vi "CAN_Command Ford.vi"(5 "CAN Command":string, 6 "ID Response":string="18DAF255", 7 "Numeric Request":u32 format="%x", 8 "ID Request":string="18DA55F2", 9 "Read":refnum<k21>, 10 "Write":refnum<k21>) -> (0 "Data String":string, 1 "ID String":string, 2 "Write out":refnum<k21>, 3 "Read out":refnum<k21>, 4 "Timestamp":timestamp)   [LabVIEW 2023]
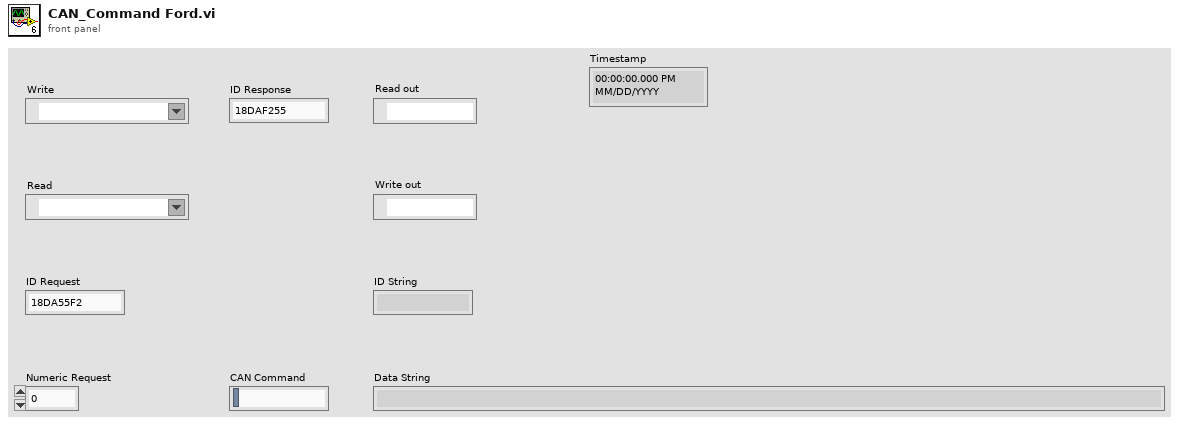
[diagram p1: front panel]
types:
  T1 = typedef "XNET Frame CAN.ctl" = cluster{"timestamp":timestamp, "payload":u8[], "identifier":u32, "type":T2, "extended?":bool, "echo?":bool}
  T2 = typedef "XNET Frame Type CAN.ctl" = u8
  T3 = cluster{"data[0]":T1, "data[1]":T1, "data[2]":T1, "data[3]":T1, "data[4]":T1, "data[5]":T1, "data[6]":T1, "data[7]":T1, "data[8]":T1}
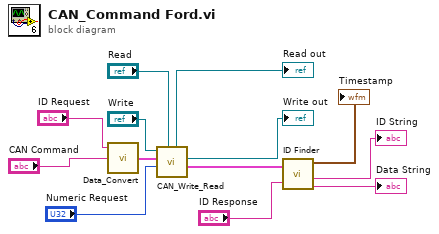
[diagram p0: block diagram]
diagram:
  n1 = call "Data_Convert.vi"("string"="CAN Command", "ID"="ID Request") -> ("CAN frame"=w10:T1)  [unwired: 1 in]
  n2 = call "CAN_Write_Read.vi"("Read In"="Read", "Numeric Request"="Numeric Request", "CAN frame"=w10, "Write In"="Write") -> ("cluster"=w11:T3, "Write Out"=→"Write out":refnum<k21>, "Read Out"=→"Read out":refnum<k21>)  [unwired: 1 in, 2 out]
  n3 = call "ID Finder.vi"("cluster"=w11, "ID ESPERADO STRING"="ID Response") -> ("Timestamp"=→"Timestamp":timestamp, "ID String"=→"ID String":string, "Data String"=→"Data String":string)  [unwired: 3 out]
